vi "2D Zero-Clean.vi"(1 "2D array input":sgl[][](array[numeric])) -> (0 "2D array output":sgl[][](array[numeric]))   [LabVIEW 2010]
doc: "Removes 0's from a 2D array using the first col"
panel:
  # "Takes a 2D array, searches the first col \nremoves any 0 values and the corresponding\nvalue form the second col"
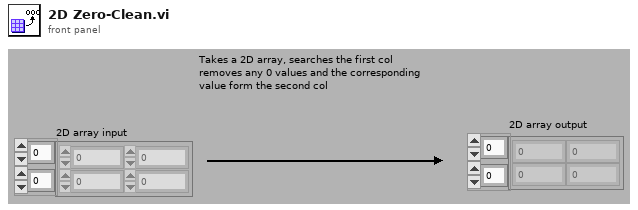
[diagram p1: front panel]
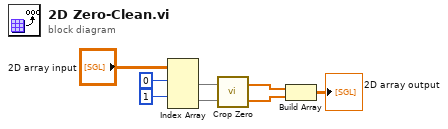
[diagram p0: block diagram]
diagram:
  n1 = Index Array(array="2D array input", index (row) #1=0, index (row) #2=1) -> (element #1=w7:sgl[], element #2=w6:sgl[])  [unwired: 2 in]
  n2 = call "Crop Zero.vi"("Paired data"=w6, "Search data"=w7) -> ("Paired data out"=w4:sgl[], "Searched data out"=w5:sgl[])
  n3 = Build Array(w5, w4) -> (→"2D array output":sgl[][])
